vi "Initialize NI-SWITCH Engine.vi"(8 "error in (no error)":errorcluster, 11 "Device Ref in":T2 format="%.0x") -> (0 "error out":errorcluster, 1 "NI-SWITCH Consumer":refnum<class "NI-SWITCH Consumer.lvclass">, 2 "FIFO Indices":T1, 3 "Device Ref out":T2 format="%.0x")   [LabVIEW 2019, in "NI-SWITCH Engine.lvlib"]
uses:
  NI-SWITCH Engine.lvlib
  <vilib>/NI VeriStand/Custom Device API/Custom Device Item Ref.ctl
  Shared/FIFO Indices.ctl
  Includes/NISWITCHMessaging.lvlibp/NI-SWITCH Consumer/NI-SWITCH Consumer.lvclass
  Shared/Compiled.Settings.ctl
  Shared/Communication Configuration.ctl
  Shared/Driver Configuration.ctl
  Includes/CDMessaging.lvlibp/Message Queue/Message Queue/Message Queue.lvclass
  C:/Dev/GitHub/niveristand-routing-and-faulting-custom-device/Includes/CDMessaging.lvlibp/Message Queue/Abstract Message Queue/Abstract Message Queue.lvclass
  Includes/NISWITCHMessaging.lvlibp/NI-SWITCH Init Parameters/NI-SWITCH Init Parameters.lvclass
  C:/Dev/GitHub/niveristand-routing-and-faulting-custom-device/Includes/CDMessaging.lvlibp/Parameters/Abstract Init Parameters/Abstract Init Parameters.lvclass
  C:/Dev/GitHub/niveristand-routing-and-faulting-custom-device/Includes/CDMessaging.lvlibp/Switch/Abstract Switch Init Parameters/Abstract Switch Init Parameters.lvclass
  Shared/Constants.vi
  <vilib>/NI VeriStand/Custom Device API/Get Item Property (Variant).vi
  <vilib>/NI VeriStand/Custom Device API/Custom Device API.lvlib
  Shared/NI-SWITCH Shared.lvlib
  Includes/CDMessaging.lvlibp/Consumer/Abstract Consumer/Abstract Consumer.lvclass
  C:/Dev/GitHub/niveristand-routing-and-faulting-custom-device/Includes/CDMessaging.lvlibp/Consumer/Abstract Consumer/Abstract Consumer.lvclass
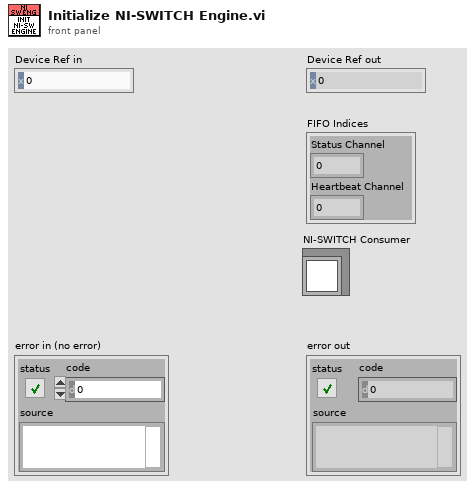
[diagram p1: front panel]
types:
  T1 = typedef "NI-SWITCH Shared.lvlib/FIFO Indices.ctl" = cluster{"Status Channel":i32, "Heartbeat Channel":i32}
  T2 = typedef "Custom Device API.lvlib/Custom Device Item Ref.ctl" = u64
  T3 = typedef "NI-SWITCH Shared.lvlib/Compiled.Settings.ctl" = cluster{"Custom Device Name":string, "Communication Configuration":T4, "Driver Configuration":T5, "FIFO Indices":T1}
  T4 = typedef "NI-SWITCH Shared.lvlib/Communication Configuration.ctl" = cluster{"Consumer Queue Name":string}
  T5 = typedef "NI-SWITCH Shared.lvlib/Driver Configuration.ctl" = cluster{"Topology":string, "Resource":string, "Source Channels":string[], "Configuration Channels":string[]}
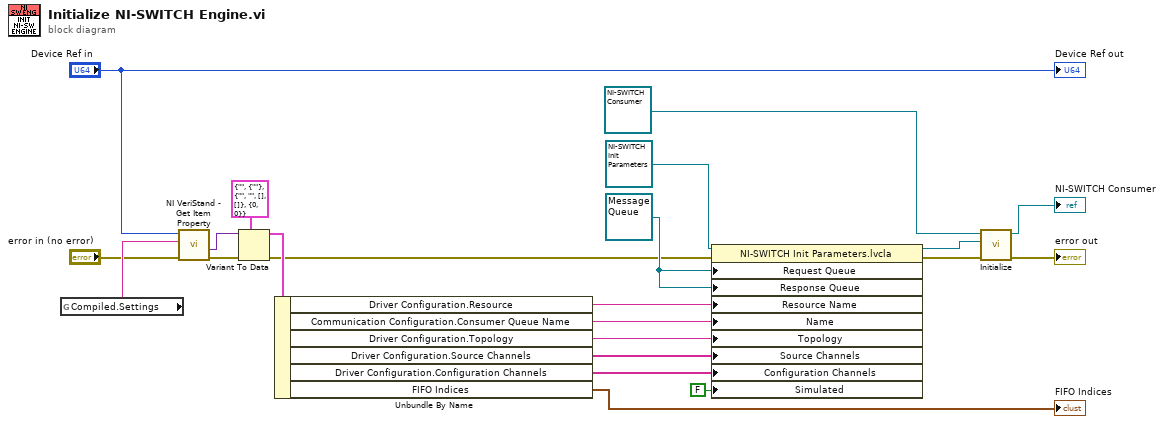
[diagram p0: block diagram]
diagram:
  w18 = refnum<class "Message Queue.lvclass"> refnum ("Request Queue")
  n1 = global read "Constants.vi" "Compiled.Settings"() -> (w22:string)
  n2 = call-poly <vilib>:"NI VeriStand - Get Item Property.vi"("error in (no error)"="error in (no error)", "Property Name"=w22, "Item Ref in"="Device Ref in") -> ("error out"=w21:errorcluster, "Value"=w20:variant)  [unwired: 5 in, 2 out]
  n3 = Variant To Data(error in=w21, type=T3 {"Custom Device Name"="", "Communication Configuration"={"Consumer Queue Name"=""}, "Driver Configuration"={"Topology"="", "Resource"="", "Source Channels"=[], "Configuration Channels"=[]}, "FIFO Indices"={"Status Channel"=0, "Heartbeat Channel"=0}} ("Compiled.Settings"), Variant=w20) -> (data=w16:T3, error out=w7:errorcluster)
  n4 = Unbundle By Name(w16) -> ("Driver Configuration.Resource"=w1:string, "Communication Configuration.Consumer Queue Name"=w5:string, "Driver Configuration.Topology"=w15:string, "Driver Configuration.Source Channels"=w9:string[], "Driver Configuration.Configuration Channels"=w8:string[], "FIFO Indices"=→"FIFO Indices":T1)
  n5 = property class="NI-SWITCH Init Parameters.lvcla"(reference=refnum<class "NI-SWITCH Init Parameters.lvclass"> refnum ("NISWITCHMessaging.lvlibp:NI-SWITCH Init Parameters.lvclass"), error in=w7, "Request Queue"=w18, "Response Queue"=w18, "Resource Name"=w1, "Name"=w5, "Topology"=w15, "Source Channels"=w9, "Configuration Channels"=w8, "Simulated"=FALSE) -> (reference out=w12:refnum<class "NI-SWITCH Init Parameters.lvclass">, error out=w14:errorcluster)
  n6 = call "Initialize.vi"("error in (no error)"=w14, "Parameters in"=w12, "Abstract Consumer in"=refnum<class "NI-SWITCH Consumer.lvclass"> refnum ("NISWITCHMessaging.lvlibp:NI-SWITCH Consumer.lvclass")) -> ("error out"=→"error out":errorcluster, "Abstract Consumer out"=→"NI-SWITCH Consumer":refnum<class "NI-SWITCH Consumer.lvclass">)  [unwired: 7 in]
  "Device Ref out" <- "Device Ref in"
